vi "notes denomination.vi"() -> ()   [LabVIEW 2020]
panel:
  out "Array":string[](array[string])
  in  "Numeric":dbl
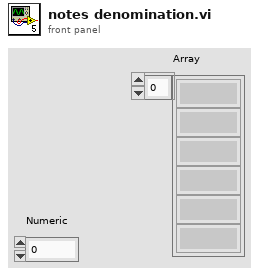
[diagram p1: front panel]
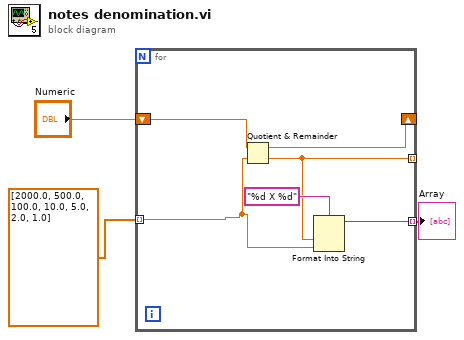
[diagram p0: block diagram]
diagram:
  n1 = for {
    tunnel: dbl[] [2000.0, 500.0, 100.0, 10.0, 5.0, 2.0, 1.0] ("Array") -> [w5] mode=indexing
    shift-right: [w8] -> _
    shift-left: "Numeric" -> [w9]
    tunnel: [w6] -> _ mode=indexing
    tunnel: [w4] -> w1 mode=indexing
    n2 = Quotient & Remainder(x=w9, y=w5) -> (x-y*floor(x/y)=w8:dbl, floor(x/y)=w6:dbl)
    n3 = Format Into String "Format Into String"(format string="%d X %d", w6, w5) -> (resulting string=w4:string)  [unwired: 2 in, 1 out]
  }
  "Array" <- w1
